vi "niRFUtil MASMT FIR Filter (SGL).vi"(7 "continue?":bool, 8 "error in (no error)":errorcluster, 10 "FIR Coefficients":sgl[](array[numeric]), 11 "X":sgl[](array[numeric])) -> (0 "error out":errorcluster, 3 "Filtered X":sgl[](array[numeric]))   [LabVIEW 2015, in "niRFUtil.lvlib"]
doc: "Filters the input sequence <B>X</B> using the direct-form FIR filter specified by <B>FIR Coefficients</B>."
uses:
  niRFUtil.lvlib
  Utilities/niRFMASMT_FFT.dll
panel:
  out "bWorkH":sgl[](array[numeric])
  out "aWorkH":sgl[](array[numeric])
  out "xWorkH":sgl[](array[numeric])
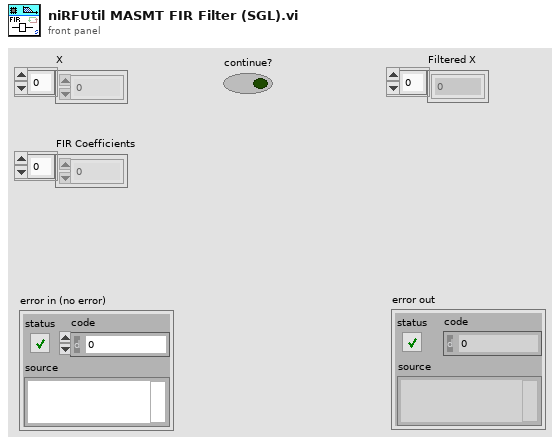
[diagram p1: front panel]
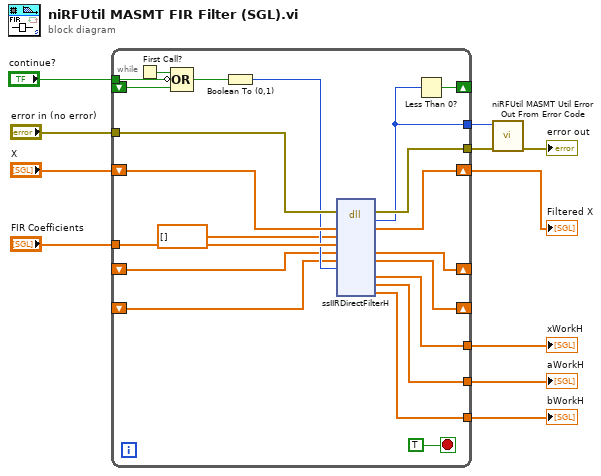
[diagram p0: block diagram]
diagram:
  n1 = while {
    tunnel: "FIR Coefficients" -> [w30]
    tunnel: [w15] -> w2
    tunnel: "error in (no error)" -> [w29]
    tunnel: [w27] -> w7
    tunnel: "continue?" -> [w24]
    tunnel: [w22] -> w5
    tunnel: [w21] -> w4
    shift-right: [w26] -> _
    shift-left: _ -> [w20]
    shift-right: [w19] -> _
    shift-left: _ -> [w12]
    shift-right: [w18] -> _
    shift-left: _ -> [w17]
    tunnel: [w14] -> w1
    shift-right: [w31] -> w10
    shift-left: "X" -> [w32]
    stop <- TRUE stop-if-true
    n2 = First Call?() -> (First Call?: T/F=w25:bool)
    n3 = Compound Arithmetic op=OR(w25, invert w24, w17) -> (w23:bool)
    n4 = Boolean To (0,1)(Boolean=w23) -> (0, 1=w28:i16)
    n5 = dll-call lib="C:/Perforce/semoore-sales/Customers/NATI-3813/Noise Floor/LV Filters/ParallelComplexFilterRFUtil/niRFUtil/MASMT/Utilities/niRFMASMT_FFT.*" fn="ssIIRDirectFilterH"(error in=w29, "xH"=w32, "aH"=sgl[] [], "bH"=w30, "x1H"=w12, "y1H"=w20, "reset"=w28) -> (error out=w15:errorcluster, "return type"=w14:i32, "xH"=w31:sgl[], "x1H"=w19:sgl[], "y1H"=w26:sgl[], "xWorkH"=w27:sgl[], "aWorkH"=w22:sgl[], "bWorkH"=w21:sgl[])  [unwired: 8 in, 1 out]
    n6 = Less Than 0?(x=w14) -> (x < 0?=w18:bool)
  }
  "Filtered X" <- w10
  "xWorkH" <- w7
  "aWorkH" <- w5
  "bWorkH" <- w4
  n7 = call "niRFUtil MASMT Util Error Out From Error Code.vi"("error in (no error)"=w2, "error code"=w1) -> ("error out"=→"error out":errorcluster)  [unwired: 9 in]
